vi "run_code.vi"   [LabVIEW 2013]
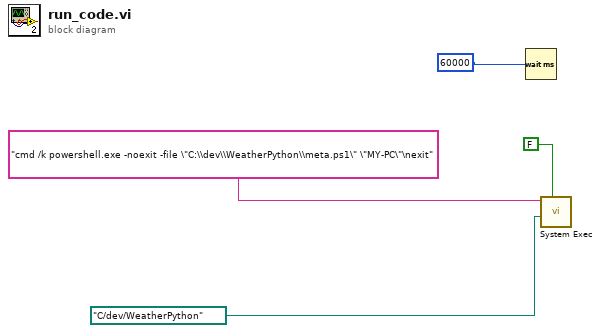
[diagram p0: block diagram]
diagram:
  n1 = Wait (ms)(milliseconds to wait=60000) -> ()  [unwired: 1 out]
  n2 = call <vilib>:"System Exec.vi"("wait until completion? (T)"=FALSE, "working directory"=path "C:/dev/WeatherPython", "command line"="cmd /k powershell.exe -noexit -file \"C:\\dev\\WeatherPython\\meta.ps1\" \"MY-PC\"\nexit") -> ()  [unwired: 5 in, 4 out]
